vi "Set Marker Mode.vi"(8 "error in (no error)":errorcluster, 10 "Marker Mode (0: Sine Wave)":u32(ring) items=["Sine Wave", "Triangular / Sawtooth Pulse", "Square Wave (50 %)", "Square Wave (20 %)"], 11 "VISA resource name":refnum<visa-resource-name>) -> (0 "error out":errorcluster, 3 "VISA resource name out":refnum<visa-resource-name>)   [LabVIEW 2014, in "Fluke 5XXX Series Multicalibrators.lvlib"]
doc: "This VI selects the waveform for Marker scope mode.\n\nNote:\n\nThis VI is available only for instrument models 5500A and 5520A with oscilloscope option SC600 (SC1100)."
uses:
  Fluke 5XXX Series Multicalibrators.lvlib
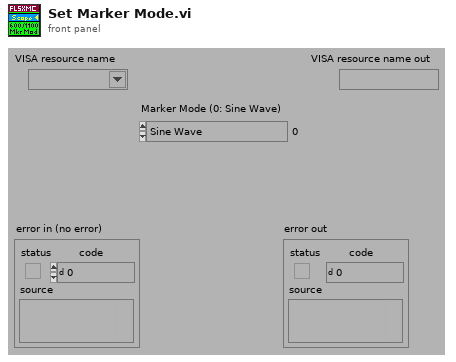
[diagram p1: front panel]
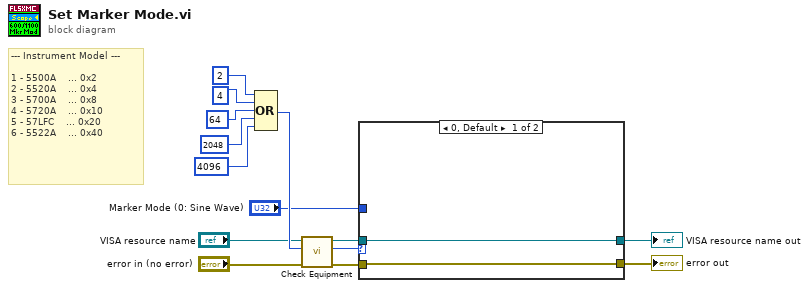
[diagram p0: block diagram]
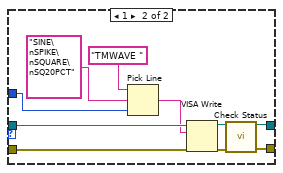
[diagram p2: hidden frame]
diagram:
  # "--- Instrument Model ---\n\n1 - 5500A    ... 0x2\n2 - 5520A    ... 0x4\n3 - 5700A    ... 0x8\n4 - 5720A    ... 0x10\n5 - 57LFC    ... 0x20\n6 - 5522A    ... 0x40"
  n1 = Compound Arithmetic op=OR(2 ("Numeric"), 4 ("Numeric"), 64 ("Numeric"), 2048 ("Numeric"), 4096 ("Numeric")) -> (w8:i32)
  n2 = call "Check Equipment.vi"("error in (no error)"="error in (no error)", "Bit Mask"=w8, "VISA resource name"="VISA resource name") -> ("error out"=w11:errorcluster, "Present?"=w10:u32, "VISA resource name out"=w9:refnum<visa-resource-name>)  [unwired: 6 in]
  n3 = case shown="0, Default" w10 {
    tunnel: [w15 w18] -> w5
    tunnel: w11 -> [w16 w24]
    tunnel: w9 -> [w15 w23]
    tunnel: [w16 w21] -> w6
    tunnel: "Marker Mode (0: Sine Wave)" -> [_ w17]
    frame 0, Default {
    }
    frame 1 {
      n4 = Pick Line(string ("")="TMWAVE " ("Reset Command"), multi-line string="SINE\nSPIKE\nSQUARE\nSQ20PCT", line index=w17) -> (output string=w22:string)
      n5 = VISA Write(VISA resource name=w23, write buffer=w22, error in (no error)=w24) -> (VISA resource name out=w19:refnum<visa-resource-name>, error out=w20:errorcluster)  [unwired: 1 out]
      n6 = call "Check Status.vi"("VISA resource name"=w19, "error in (no error)"=w20) -> ("VISA resource name out"=w18:refnum<visa-resource-name>, "error out"=w21:errorcluster)  [unwired: 12 in]
    }
  }
  "VISA resource name out" <- w5
  "error out" <- w6
